vi "счётчик.vi"(3 "T":bool) -> (0 "x1":bool, 1 "x0":bool)   [LabVIEW 2012]
panel:
  in  "Boolean":bool
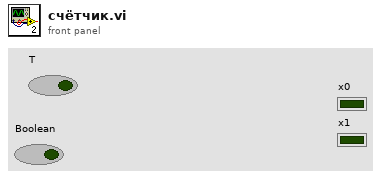
[diagram p1: front panel]
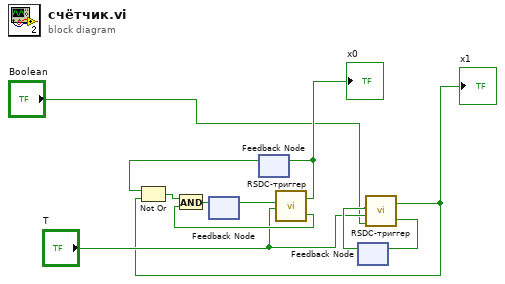
[diagram p0: block diagram]
diagram:
  n1 = feedback #1() -> (w8:bool)  [unwired: 1 in]
  n2 = feedback #2() -> (w11:bool)  [unwired: 1 in]
  n3 = call "RSDC-триггер.vi"("C"="T", "D"=w8) -> ("not Q"=w6:bool, "Q"=w5:bool)  [unwired: 2 in]
  "x0" <- w5
  n4 = feedback-in #2(w5) -> ()
  n5 = feedback #3() -> (w10:bool)  [unwired: 1 in]
  n6 = call "RSDC-триггер.vi"("S"="Boolean", "C"="T", "D"=w10) -> ("not Q"=w2:bool, "Q"=w1:bool)  [unwired: 1 in]
  "x1" <- w1
  n7 = Not Or(1:w1, 2:w11) -> (0:w9:bool)
  n8 = And(x=w9, y=w6) -> (x .and. y?=w7:bool)
  n9 = feedback-in #1(w7) -> ()
  n10 = feedback-in #3(w2) -> ()
